vi "Actor Core.vi"(8 "error in":errorcluster, 11 "Login View In":refnum<class "Login View.lvclass">) -> (0 "error out":errorcluster, 3 "Actor out":refnum<class "Actor.lvclass">)   [LabVIEW 2017, in "Login View.lvlib" / "Login View.lvclass"]
doc: "(<B>Filename</B>: Actor Framework.lvlib:Actor.lvclass:Actor Core.vi)\n\nReceives messages to the actor, reacts to them, and initiates any error handling that may shut the actor down.\n\nDescendant classes may override this VI to append parallel tasks for the actor to complete while it handles messages. Overrides use the Call Parent Method node.\n\n<License>\nCopyright © 2017 Composed Systems, LLC | All rights reserved\nwww.composed.io\n\nAuthor: Ethan Stern <ethan.stern@composed.io>\n\nThis software is provided \"AS IS\" WITHOUT WARRANTIES, either express or implied, AND IS FOR EDUCATIONAL PURPOSES ONLY.\n</License>"
uses:
  Login View.lvclass
  <vilib>/gpm_packages/@cs/mva-viewable/Source/ActorEvents/IEventAggregator/IEventAggregator.lvclass
  <vilib>/event_ctls.llb/lveventtype.ctl
  <vilib>/gpm_packages/@cs/mva-core/Source/IObserver/IObserver/IObserver.lvclass
  <vilib>/gpm_packages/@cs/mva-core/Source/SubscriptionPolicy/BasicSubscription/BasicSubscription.lvclass
  Login View Messages/Login Failure Msg/Login Failure Msg.lvclass
  User Manager Model/Type Definitions/Successful Login Information.ctl
  User Manager Model/Type Definitions/User Manager Application Types.lvlib
  Login View Messages/Login Successful Msg/Login Successful Msg.lvclass
  User Manager Model/Type Definitions/User Levels.ctl
  C:/Program Files/National Instruments/LabVIEW 2017/vi.lib/gpm_packages/@cs/mva-viewable/Source/IViewable/IViewable/IViewable.lvclass
  C:/Program Files/National Instruments/LabVIEW 2017/vi.lib/gpm_packages/@cs/mva-viewable/Source/ActorEvents/IEventAggregator/IEventAggregator.lvclass
  C:/Program Files/National Instruments/LabVIEW 2017/vi.lib/gpm_packages/@cs/mva-core/Source/IObserver/IObserver/IObserver.lvclass
  C:/Program Files/National Instruments/LabVIEW 2017/vi.lib/ActorFramework/Actor/Actor.lvclass
  <vilib>/gpm_packages/@cs/mva-viewable/Source/IViewable/IViewable/IViewable.lvclass
  C:/Program Files/National Instruments/LabVIEW 2017/vi.lib/gpm_packages/@cs/mva-core/Source/IMediator/ISubscriptionPolicy/ISubscriptionPolicy.lvclass
  C:/Program Files/National Instruments/LabVIEW 2017/vi.lib/gpm_packages/@cs/transport/Source/Concrete/ActorMessageTransport/Notification Msg/Notification Msg.lvclass
  C:/Program Files/National Instruments/LabVIEW 2017/vi.lib/gpm_packages/@cs/actor-framework-messages/Source/RoundTripMessage/RoundTripMessage.lvclass
  C:/Program Files/National Instruments/LabVIEW 2017/vi.lib/ActorFramework/Message/Message.lvclass
  <vilib>/ActorFramework/Actor/Actor.lvclass
  User Manager Model/Type Definitions/Credentials.ctl
panel:
  in  "Credentials":T1
  in  "Login Response":string
  in  "Log In":bool
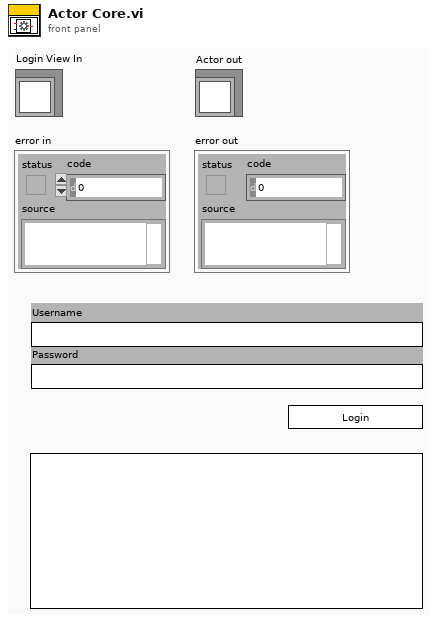
[diagram p1: front panel]
types:
  T1 = typedef "User Manager Application Types.lvlib/Credentials.ctl" = cluster{"Username":string, "Password":string}
  T2 = typedef "lveventtype.ctl" = enum32{"Null", "Timeout", "Annotation Menu Selection", "Annotation Menu Selection?", "App Instance Close", "App Instance Close?", "Autoscale Range Change", "Bookmark Info Change", "Cell Edit", "Cell Edit?", "Cursor Grab", "Cursor Grab?", "Cursor Menu Selection", "Cursor Menu Selection?", "Cursor Move", "Cursor Release", "Data Change", "Direction Change", "Display State Change", "Drag Ended", "Drag Enter", "Drag Leave", "Drag Over", "Drag Source Update", "Drag Starting", "Drag Starting?", "Drop", "Exec State Change", "Key Down", "Key Down?", "Key Repeat", "Key Repeat?", "Key Up", "Listbox Double Click", "Menu Activation?", "Menu Selection (App)", "Menu Selection? (App)", "Menu Selection (User)", "Mouse Down", "Mouse Down?", "Mouse Enter", "Mouse Leave", "Mouse Move", "Mouse Up", "Mouse Wheel", "NI Security User Change (App)", "Pane Size", "Panel Close", "Panel Close?", "Panel Resize", "Plot Attribute Change", "Scale Range Change", "Shortcut Menu Activation?", "Shortcut Menu Selection (App)", "Shortcut Menu Selection? (App)", "Shortcut Menu Selection (User)", "Tree Double Click", "Tree Drag", "Tree Drag?", "Tree Drop", "Tree Drop?", "Tree Item Close", "Tree Item Close?", "Tree Item Open", "Tree Item Open?", "User Event", "Value Change"}
  T3 = typedef "User Manager Application Types.lvlib/Successful Login Information.ctl" = cluster{"Username":string, "User Level":T4, "User Levels In This Society":T4[]}
  T4 = typedef "User Manager Application Types.lvlib/User Levels.ctl" = cluster{"Rank":i32, "Title":string}
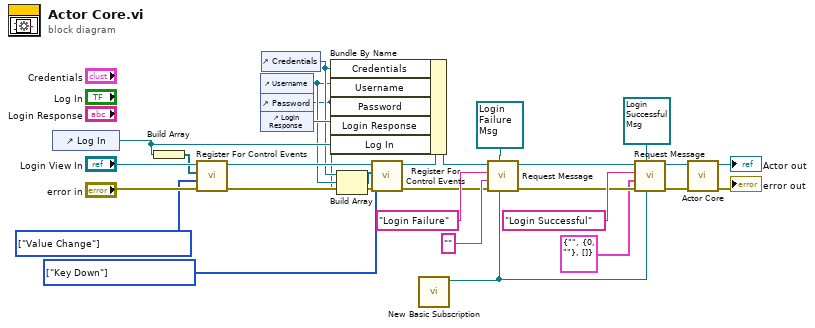
[diagram p0: block diagram]
diagram:
  w5 = T2[] [enum."Key Down"] items=["Null", "Timeout", "Annotation Menu Selection", "Annotation Menu Selection?", "App Instance Close", "App Instance Close?", "Autoscale Range Change", "Bookmark Info Change", "Cell Edit", "Cell Edit?", "Cursor Grab", "Cursor Grab?", "Cursor Menu Selection", "Cursor Menu Selection?", "Cursor Move", "Cursor Release", "Data Change", "Direction Change", "Display State Change", "Drag Ended", "Drag Enter", "Drag Leave", "Drag Over", "Drag Source Update", "Drag Starting", "Drag Starting?", "Drop", "Exec State Change", "Key Down", "Key Down?", "Key Repeat", "Key Repeat?", "Key Up", "Listbox Double Click", "Menu Activation?", "Menu Selection (App)", "Menu Selection? (App)", "Menu Selection (User)", "Mouse Down", "Mouse Down?", "Mouse Enter", "Mouse Leave", "Mouse Move", "Mouse Up", "Mouse Wheel", "NI Security User Change (App)", "Pane Size", "Panel Close", "Panel Close?", "Panel Resize", "Plot Attribute Change", "Scale Range Change", "Shortcut Menu Activation?", "Shortcut Menu Selection (App)", "Shortcut Menu Selection? (App)", "Shortcut Menu Selection (User)", "Tree Double Click", "Tree Drag", "Tree Drag?", "Tree Drop", "Tree Drop?", "Tree Item Close", "Tree Item Close?", "Tree Item Open", "Tree Item Open?", "User Event", "Value Change"] ("Registration Types")
  w24 = T2[] [enum."Value Change"] items=["Null", "Timeout", "Annotation Menu Selection", "Annotation Menu Selection?", "App Instance Close", "App Instance Close?", "Autoscale Range Change", "Bookmark Info Change", "Cell Edit", "Cell Edit?", "Cursor Grab", "Cursor Grab?", "Cursor Menu Selection", "Cursor Menu Selection?", "Cursor Move", "Cursor Release", "Data Change", "Direction Change", "Display State Change", "Drag Ended", "Drag Enter", "Drag Leave", "Drag Over", "Drag Source Update", "Drag Starting", "Drag Starting?", "Drop", "Exec State Change", "Key Down", "Key Down?", "Key Repeat", "Key Repeat?", "Key Up", "Listbox Double Click", "Menu Activation?", "Menu Selection (App)", "Menu Selection? (App)", "Menu Selection (User)", "Mouse Down", "Mouse Down?", "Mouse Enter", "Mouse Leave", "Mouse Move", "Mouse Up", "Mouse Wheel", "NI Security User Change (App)", "Pane Size", "Panel Close", "Panel Close?", "Panel Resize", "Plot Attribute Change", "Scale Range Change", "Shortcut Menu Activation?", "Shortcut Menu Selection (App)", "Shortcut Menu Selection? (App)", "Shortcut Menu Selection (User)", "Tree Double Click", "Tree Drag", "Tree Drag?", "Tree Drop", "Tree Drop?", "Tree Item Close", "Tree Item Close?", "Tree Item Open", "Tree Item Open?", "User Event", "Value Change"] ("Registration Types")
  n1 = control-ref of="Log In"() -> (w25:refnum<vi>)
  n2 = Build Array(w25) -> (w6:refnum<vi>[])
  n3 = call <vilib>:"Register For Control Events.vi"("error in (no error)"="error in", "Registration Types"=w24, "Control Refnums"=w6, "IEventAggregator In"="Login View In") -> ("error out"=w9:errorcluster, "IEventAggregator Out"=w10:refnum<class "Login View.lvclass">)  [unwired: 6 in]
  n4 = control-ref of="Username"() -> (w2:refnum<vi>)
  n5 = control-ref of="Password"() -> (w1:refnum<vi>)
  n6 = control-ref of="Login Response"() -> (w19:refnum<vi>)
  n7 = control-ref of="Credentials"() -> (w4:refnum<vi>)
  n8 = Build Array(w4, w2, w1) -> (w3:refnum<vi>[])
  n9 = call <vilib>:"Register For Control Events.vi"("error in (no error)"=w9, "Registration Types"=w5, "Control Refnums"=w3, "IEventAggregator In"=w10) -> ("error out"=w7:errorcluster, "IEventAggregator Out"=w8:refnum<class "Login View.lvclass">)  [unwired: 6 in]
  n10 = Bundle By Name(cluster=w8, "Credentials"=w4, "Username"=w2, "Password"=w1, "Login Response"=w19, "Log In"=w25) -> (w23:refnum<class "Login View.lvclass">)
  n11 = call <vilib>:"New Basic Subscription.vi"() -> ("BasicSubscription Out"=w11:refnum<class "BasicSubscription.lvclass">)  [unwired: 11 in]
  n12 = call <vilib>:"Request Message.vi"("Configured SubscriptionPolicy"=w11, "Desired Notification Msg"=refnum<class "Login Failure Msg.lvclass"> refnum ("Login View.lvlib:Login Failure Msg.lvclass"), "error in (no error)"=w7, "Data Type"="", "Datum Name"="Login Failure", "IObserver in"=w23) -> ("error out"=w15:errorcluster, "IObserver out"=w16:refnum<class "Login View.lvclass">)  [unwired: 3 in, 1 out]
  n13 = call <vilib>:"Request Message.vi"("Configured SubscriptionPolicy"=w11, "Desired Notification Msg"=refnum<class "Login Successful Msg.lvclass"> refnum ("Login View.lvlib:Login Successful Msg.lvclass"), "error in (no error)"=w15, "Data Type"=T3 {"Username"="", "User Level"={"Rank"=0, "Title"=""}, "User Levels In This Society"=[]}, "Datum Name"="Login Successful", "IObserver in"=w16) -> ("error out"=w17:errorcluster, "IObserver out"=w12:refnum<class "Login View.lvclass">)  [unwired: 3 in, 1 out]
  n14 = call-parent "Actor Core.vi"("error in"=w17, "IViewable In"=w12) -> ("error out"=→"error out":errorcluster, "Actor out"=→"Actor out":refnum<class "Actor.lvclass">)  [unwired: 8 in]
